vi "水样测试.vi"(11 "数据标记表":string(combo)="N") -> ()   [LabVIEW 2016, in "斯坦道多参数.lvlib"]
panel:
  out "运行状态":u16(ring) items=["空闲", "水样测试", "标样核查"]
  out "多参数运行日志":string
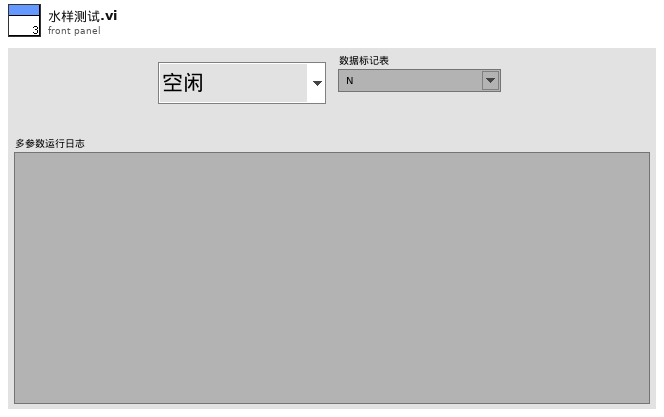
[diagram p1: front panel]
types:
  T1 = typedef "集成多参数单参数字段定义.ctl" = cluster{"时间":timestamp, "测量模式":string, "数据类型":string, "检测值":sgl, "单位":string, "数据标识":string, "信号值":sgl, "标样参考值":sgl, "因子编码":string, "探头温度":sgl, "LastTime":timestamp}
  T2 = cluster{"水温":bool, "pH":bool, "DO":bool, "DOper":bool, "电导率":bool, "ORP":bool, "浊度":bool, "叶绿素a":bool, "藻密度":bool, "COD":bool, "DO2":bool, "DOper":bool, "氯化物":bool, "氨氮":bool, "水中油":bool}
  T3 = cluster{"ph":bool, "DO":bool, "Cond":bool, "Turb":bool, "叶绿素a":bool, "藻密度":bool, "ORP":bool, "cod":bool, "DO2":bool, "氯化物":bool, "氨氮":bool, "水中油":bool}
  T4 = cluster{"温度测量值":sgl, "测量值":sgl, "温度偏移修正值":sgl, "信号值":sgl, "数据标识":string}
  T5 = cluster{"温度测量值":sgl, "DO%":sgl, "DOmg/L":sgl, "温度偏移修正值":sgl, "数据标识mg/L":string, "数据标识%":string}
  T6 = cluster{"CH":u16, "监测值":dbl, "信号值":sgl, "数据标识":string}
  T7 = cluster{"水样数据时间":timestamp, "水温":dbl, "pH":dbl, "DO":dbl, "DOper":dbl, "电导率":dbl, "ORP":dbl, "浊度":dbl, "叶绿素a":dbl, "藻密度":dbl, "COD":dbl, "DO2":dbl, "DO2per":dbl, "氯化物":dbl, "氨氮":dbl, "水中油":dbl}
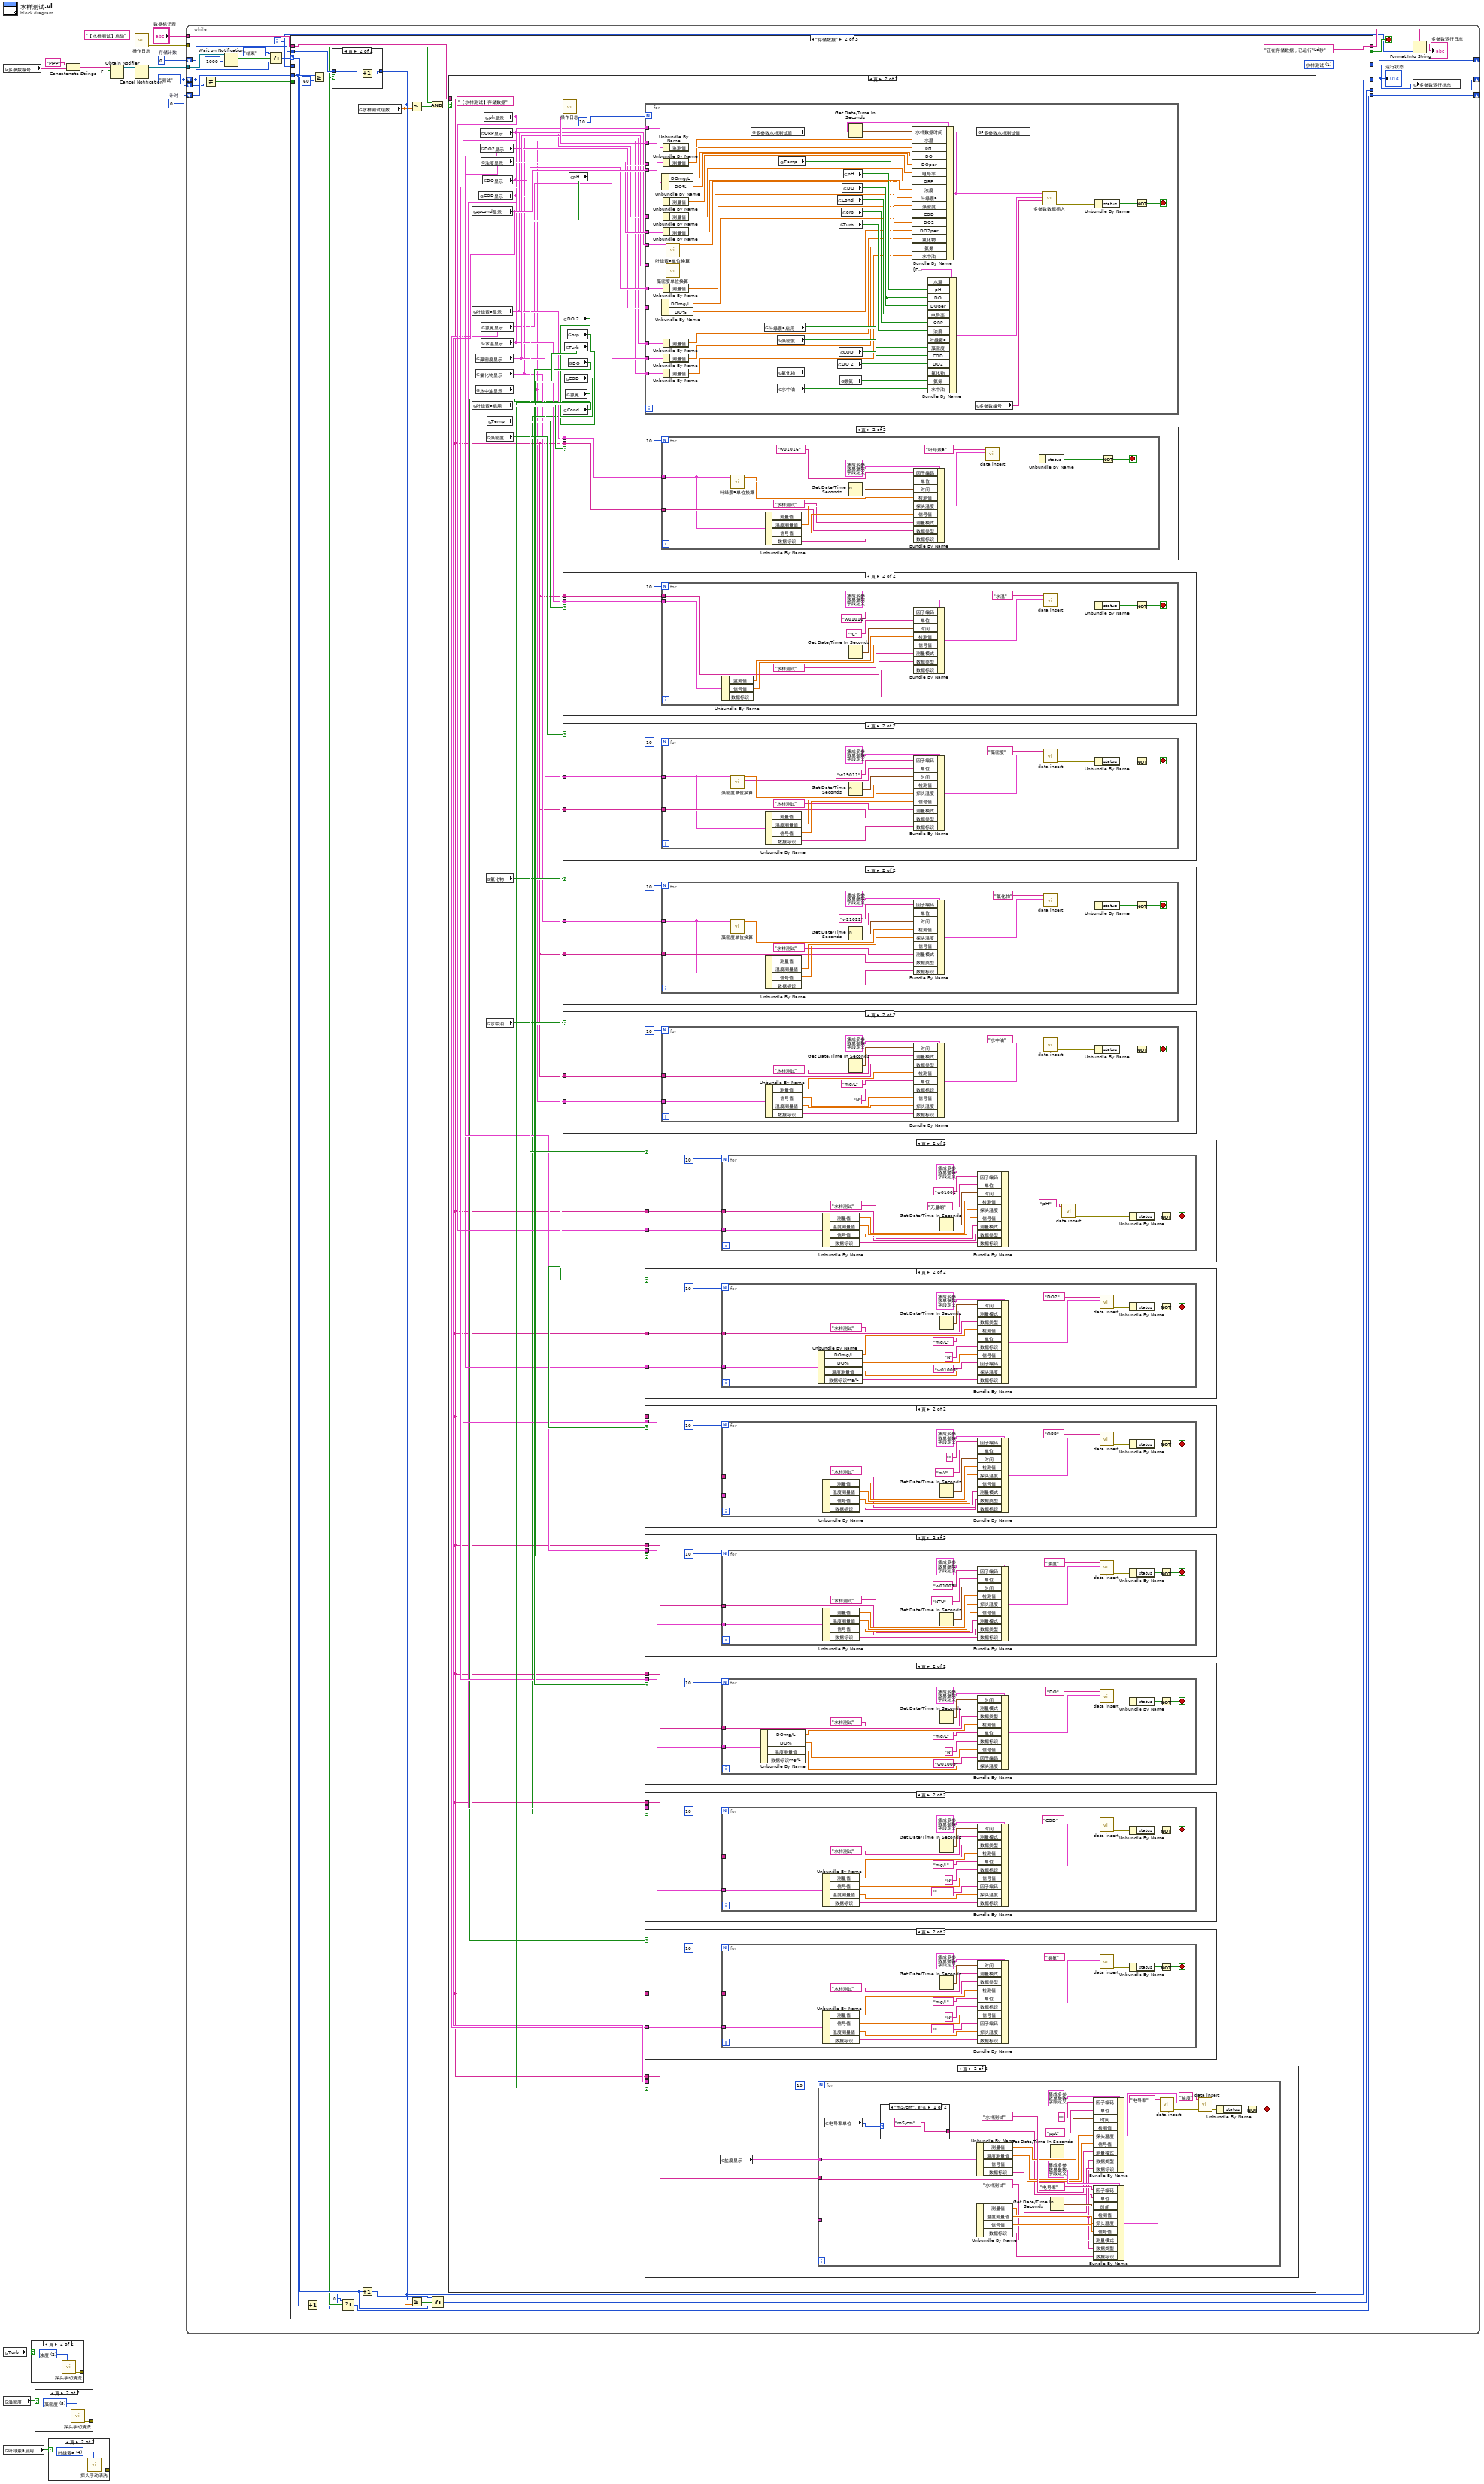
[diagram p0: block diagram]
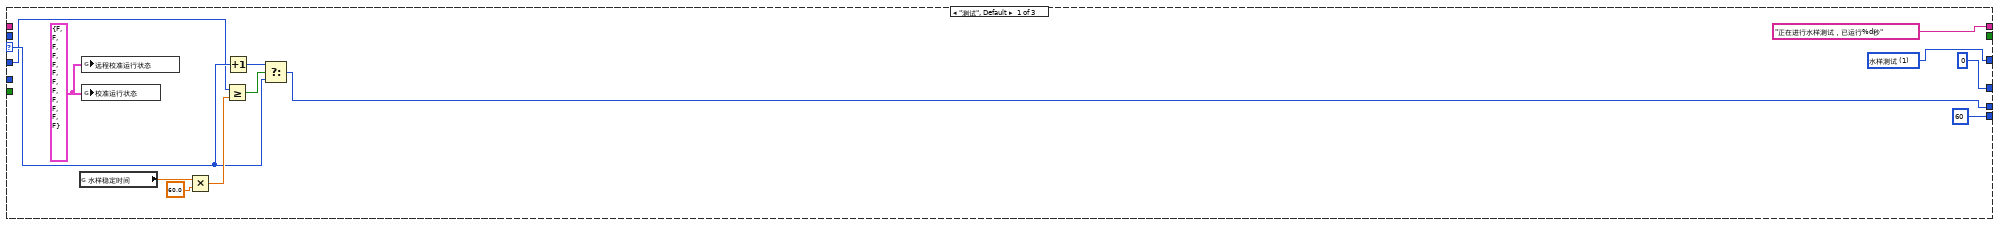
[diagram p5: hidden frame]
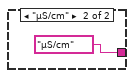
[diagram p18: hidden frame]
diagram:
  w7 = 0  # 存储计数
  w8 = 0  # 计时
  w3 = enum16{"测试", "存储数据", "结束"}."测试" ("枚举")
  n1 = global read "多参数全局变量.vi" "多参数编号"() -> (w9:string)
  n2 = global read "断电保存变量.vi" "Turb"() -> (w6:bool)
  n3 = global read "断电保存变量.vi" "藻密度"() -> (w4:bool)
  n4 = global read "断电保存变量.vi" "叶绿素a启用"() -> (w5:bool)
  n5 = case shown="真" w6 {
    tunnel: [_ w16] -> _
    frame False {
    }
    frame True {
      w17 = u16 2 items=["pH", "DO", "浊度", "电导率", "叶绿素a", "藻密度", "ORP", "DO2"] ("校准参数")
      n6 = call "探头手动清洗.vi"("校准参数"=w17) -> ("error out"=w16:errorcluster)  [unwired: 10 in]
    }
  }
  n7 = case shown="真" w4 {
    tunnel: [_ w18] -> _
    frame False {
    }
    frame True {
      w19 = u16 5 items=["pH", "DO", "浊度", "电导率", "叶绿素a", "藻密度", "ORP", "DO2"] ("校准参数")
      n8 = call "探头手动清洗.vi"("校准参数"=w19) -> ("error out"=w18:errorcluster)  [unwired: 10 in]
    }
  }
  n9 = case shown="真" w5 {
    tunnel: [_ w20] -> _
    frame False {
    }
    frame True {
      w21 = u16 4 items=["pH", "DO", "浊度", "电导率", "叶绿素a", "藻密度", "ORP", "DO2"] ("校准参数")
      n10 = call "探头手动清洗.vi"("校准参数"=w21) -> ("error out"=w20:errorcluster)  [unwired: 10 in]
    }
  }
  n11 = Concatenate Strings("MPP" ("名称（未命名）"), w9) -> (w10:string)
  n12 = Obtain Notifier(name (unnamed)=w10, notification data type=FALSE) -> (notifier out=w13:refnum<notifier>)  [unwired: 2 in, 2 out]
  n13 = call "操作日志.vi"("日志信息"="【水样测试】启动") -> ("error out"=w1:errorcluster)  [unwired: 10 in]
  n14 = Cancel Notification(0:w13) -> (8:w12:refnum<notifier>)  [unwired: 1 in, 2 out]
  n15 = while {
    shift-right: [w26] -> _
    shift-left: w3 -> [w24]
    tunnel: w12 -> [w37]
    tunnel: "数据标记表" -> [w32]
    shift-right: [w28] -> _
    shift-left: w8 -> [w30]
    shift-right: [w27] -> _
    shift-left: w7 -> [w29]
    shift-left: w3 -> [w23]
    tunnel: w1 -> [_]
    i -> [w25]
    stop <- w40 stop-if-true
    n16 = Not Equal?(x=w24, y=w23) -> (x != y?=w22:bool)
    n17 = Wait on Notification(notifier=w37, timeout in ms (-1)=1000 ("超时毫秒(-1)")) -> (notification=w35:bool)  [unwired: 2 in, 3 out]
    n18 = Select(t=enum16{"测试", "存储数据", "结束"}."结束" ("枚举"), s=w35, f=w24) -> (s? t:f=w33:enum16{"测试", "存储数据", "结束"})
    n19 = case shown="\"存储数据\"" w33 {
      selector: w33 -> [w47 w61 _]
      tunnel: [_ _ TRUE] -> w40
      tunnel: ["正在进行水样测试，已运行%d秒" ("格式字符串") "正在存储数据，已运行%d秒" ("格式字符串") "测试停止，累计运行%d秒" ("格式字符串")] -> w39
      tunnel: [w52 w66 w424] -> w31
      tunnel: w32 -> [_ w71 _]
      tunnel: w30 -> [_ w69 _]
      tunnel: w29 -> [_ w70 _]
      tunnel: [60 w54 0] -> w28
      tunnel: [0 w60 0] -> w27
      tunnel: [w45 w64 enum16{"测试", "存储数据", "结束"}."结束" ("枚举")] -> w26
      tunnel: w25 -> [w42 _ _]
      tunnel: w22 -> [_ _ w420]
      frame "测试", Default {
        w41 = T3 {"ph"=FALSE, "DO"=FALSE, "Cond"=FALSE, "Turb"=FALSE, "叶绿素a"=FALSE, "藻密度"=FALSE, "ORP"=FALSE, "cod"=FALSE, "DO2"=FALSE, "氯化物"=FALSE, "氨氮"=FALSE, "水中油"=FALSE} ("远程校准运行状态")
        w52 = u16 1 items=["空闲", "水样测试", "标样核查"] ("多参数运行状态")
        n20 = global read "断电保存变量.vi" "水样稳定时间"() -> (w51:dbl)
        n21 = global write "多参数全局变量.vi" "远程校准运行状态"(w41) -> ()
        n22 = global write "多参数全局变量.vi" "校准运行状态"(w41) -> ()
        n23 = Multiply(x=w51, y=60.0) -> (x*y=w49:dbl)
        n24 = Greater Or Equal?(x=w42, y=w49) -> (x >= y?=w48:bool)
        n25 = Increment(x=w47) -> (x+1=w46:enum16{"测试", "存储数据", "结束"})
        n26 = Select(t=w46, s=w48, f=w47) -> (s? t:f=w45:enum16{"测试", "存储数据", "结束"})
      }
      frame "存储数据" {
        w66 = u16 1 items=["空闲", "水样测试", "标样核查"] ("多参数运行状态")
        n27 = Increment(x=w69) -> (x+1=w56:i32)
        n28 = Greater Or Equal?(x=w69, y=60) -> (x >= y?=w57:bool)
        n29 = case shown="真" w57 {
          tunnel: w70 -> [w72 w74]
          tunnel: [w72 w73] -> w60
          frame False {
          }
          frame True {
            n30 = Increment(x=w74) -> (x+1=w73:i32)
          }
        }
        n31 = Select(t=0, s=w57, f=w56) -> (s? t:f=w54:i32)
        n32 = global read "断电保存变量.vi" "水样测试组数"() -> (w59:dbl)
        n33 = Increment(x=w61) -> (x+1=w62:enum16{"测试", "存储数据", "结束"})
        n34 = Less Or Equal?(x=w60, y=w59) -> (x <= y?=w65:bool)
        n35 = Greater Or Equal?(x=w60, y=w59) -> (x >= y?=w58:bool)
        n36 = And(x=w57, y=w65) -> (x .and. y?=w63:bool)
        n37 = Select(t=w62, s=w58, f=w61) -> (s? t:f=w64:enum16{"测试", "存储数据", "结束"})
        n38 = case shown="真" w63 {
          tunnel: w71 -> [_ w76]
          frame False {
          }
          frame True {
            n39 = global read "多参数全局变量.vi" "spcond显示"() -> (w94:T4)
            n40 = global read "多参数全局变量.vi" "叶绿素a显示"() -> (w88:T4)
            n41 = global read "断电保存变量.vi" "叶绿素a启用"() -> (w103:bool)
            n42 = global read "多参数全局变量.vi" "藻密度显示"() -> (w90:T4)
            n43 = global read "多参数全局变量.vi" "氯化物显示"() -> (w80:T4)
            n44 = global read "多参数全局变量.vi" "水中油显示"() -> (w75:T4)
            n45 = global read "多参数全局变量.vi" "COD显示"() -> (w85:T4)
            n46 = global read "多参数全局变量.vi" "ORP显示"() -> (w87:T4)
            n47 = global read "多参数全局变量.vi" "DO2显示"() -> (w82:T5)
            n48 = global read "多参数全局变量.vi" "浊度显示"() -> (w92:T4)
            n49 = global read "多参数全局变量.vi" "氨氮显示"() -> (w78:T4)
            n50 = global read "多参数全局变量.vi" "水温显示"() -> (w89:T6)
            n51 = global read "多参数全局变量.vi" "DO显示"() -> (w91:T5)
            n52 = global read "多参数全局变量.vi" "ph显示"() -> (w93:T4)
            n53 = global read "断电保存变量.vi" "藻密度"() -> (w97:bool)
            n54 = global read "断电保存变量.vi" "氯化物"() -> (w81:bool)
            n55 = global read "断电保存变量.vi" "水中油"() -> (w77:bool)
            n56 = global read "断电保存变量.vi" "Temp"() -> (w98:bool)
            n57 = call "操作日志.vi"("日志信息"="【水样测试】存储数据") -> ()  [unwired: 10 in, 1 out]
            n58 = global read "断电保存变量.vi" "DO 2"() -> (w83:bool)
            n59 = global read "断电保存变量.vi" "Cond"() -> (w101:bool)
            n60 = case shown="真" w103 {
              tunnel: w76 -> [_ w292]
              tunnel: w88 -> [_ w290]
              frame False {
              }
              frame True {
                n61 = for {
                  N: 10 -> [_]
                  tunnel: w292 -> [w298]
                  tunnel: w290 -> [w295]
                  stop <- w302 stop-if-true
                  n62 = call "叶绿素a单位换算.vi"("叶绿素a显示"=w295) -> ("检测值1.单位"=w294:string, "测量值"=w293:sgl)  [unwired: 8 in, 1 out]
                  n63 = Unbundle By Name(w295) -> ("温度测量值"=w308:sgl, "信号值"=w301:sgl, "数据标识"=w297:string)  [unwired: 1 out]
                  n64 = Get Date/Time In Seconds() -> (seconds since 1Jan1904=w300:timestamp)
                  n65 = Bundle By Name(cluster=T1 {"时间"=timestamp(0 s since 1904-01-01), "测量模式"="水样测试", "数据类型"="N", "检测值"=0.0, "单位"="mg/L", "数据标识"="N", "信号值"=0.0, "标样参考值"=0.0, "因子编码"="", "探头温度"=0.0, "LastTime"=timestamp(0 s since 1904-01-01)} ("data"), "因子编码"="w01016", "单位"=w294, "时间"=w300, "检测值"=w293, "探头温度"=w308, "信号值"=w301, "测量模式"="水样测试", "数据类型"=w298, "数据标识"=w297) -> (w306:T1)
                  n66 = call "data insert.vi"("data"=w306, "table in"="叶绿素a" ("table输入")) -> ("error out"=w304:errorcluster)  [unwired: 9 in]
                  n67 = Unbundle By Name(w304) -> ("status"=w303:bool)
                  n68 = Not(x=w303) -> (.not. x?=w302:bool)
                }
              }
            }
            n69 = case shown="真" w98 {
              tunnel: w76 -> [_ w404]
              tunnel: w89 -> [_ w402]
              frame False {
              }
              frame True {
                n70 = for {
                  N: 10 -> [_]
                  tunnel: w404 -> [w408]
                  tunnel: w402 -> [w407]
                  stop <- w412 stop-if-true
                  n71 = Unbundle By Name(w407) -> ("监测值"=w415:dbl, "信号值"=w410:sgl, "数据标识"=w406:string)
                  n72 = Get Date/Time In Seconds() -> (seconds since 1Jan1904=w411:timestamp)
                  n73 = Bundle By Name(cluster=T1 {"时间"=timestamp(0 s since 1904-01-01), "测量模式"="水样测试", "数据类型"="N", "检测值"=0.0, "单位"="mg/L", "数据标识"="N", "信号值"=0.0, "标样参考值"=0.0, "因子编码"="", "探头温度"=0.0, "LastTime"=timestamp(0 s since 1904-01-01)} ("data"), "因子编码"="w01010", "单位"="℃", "时间"=w411, "检测值"=w415, "信号值"=w410, "测量模式"="水样测试", "数据类型"=w408, "数据标识"=w406) -> (w418:T1)
                  n74 = call "data insert.vi"("data"=w418, "table in"="水温" ("table输入")) -> ("error out"=w414:errorcluster)  [unwired: 9 in]
                  n75 = Unbundle By Name(w414) -> ("status"=w413:bool)
                  n76 = Not(x=w413) -> (.not. x?=w412:bool)
                }
              }
            }
            n77 = case shown="真" w97 {
              tunnel: w76 -> [_ w273]
              tunnel: w90 -> [_ w271]
              frame False {
              }
              frame True {
                n78 = for {
                  N: 10 -> [_]
                  tunnel: w273 -> [w280]
                  tunnel: w271 -> [w276]
                  stop <- w281 stop-if-true
                  n79 = call "藻密度单位换算.vi"("藻密度显示"=w276) -> ("检测值1.单位"=w274:string, "测量值"=w275:sgl)  [unwired: 8 in, 1 out]
                  n80 = Unbundle By Name(w276) -> ("温度测量值"=w289:sgl, "信号值"=w282:sgl, "数据标识"=w278:string)  [unwired: 1 out]
                  n81 = Get Date/Time In Seconds() -> (seconds since 1Jan1904=w283:timestamp)
                  n82 = Bundle By Name(cluster=T1 {"时间"=timestamp(0 s since 1904-01-01), "测量模式"="水样测试", "数据类型"="N", "检测值"=0.0, "单位"="mg/L", "数据标识"="N", "信号值"=0.0, "标样参考值"=0.0, "因子编码"="", "探头温度"=0.0, "LastTime"=timestamp(0 s since 1904-01-01)} ("data"), "因子编码"="w19011", "单位"=w274, "时间"=w283, "检测值"=w275, "探头温度"=w289, "信号值"=w282, "测量模式"="水样测试", "数据类型"=w280, "数据标识"=w278) -> (w284:T1)
                  n83 = call "data insert.vi"("data"=w284, "table in"="藻密度" ("table输入")) -> ("error out"=w286:errorcluster)  [unwired: 9 in]
                  n84 = Unbundle By Name(w286) -> ("status"=w285:bool)
                  n85 = Not(x=w285) -> (.not. x?=w281:bool)
                }
              }
            }
            n86 = case shown="真" w81 {
              tunnel: w76 -> [_ w145]
              tunnel: w80 -> [_ w143]
              frame False {
              }
              frame True {
                n87 = for {
                  N: 10 -> [_]
                  tunnel: w145 -> [w154]
                  tunnel: w143 -> [w150]
                  stop <- w155 stop-if-true
                  n88 = call "藻密度单位换算.vi"("藻密度显示"=w150) -> ("检测值1.单位"=w148:string, "测量值"=w149:sgl)  [unwired: 8 in, 1 out]
                  n89 = Unbundle By Name(w150) -> ("温度测量值"=w161:sgl, "信号值"=w156:sgl, "数据标识"=w152:string)  [unwired: 1 out]
                  n90 = Get Date/Time In Seconds() -> (seconds since 1Jan1904=w157:timestamp)
                  n91 = Bundle By Name(cluster=T1 {"时间"=timestamp(0 s since 1904-01-01), "测量模式"="水样测试", "数据类型"="N", "检测值"=0.0, "单位"="mg/L", "数据标识"="N", "信号值"=0.0, "标样参考值"=0.0, "因子编码"="", "探头温度"=0.0, "LastTime"=timestamp(0 s since 1904-01-01)} ("data"), "因子编码"="w21022", "单位"=w148, "时间"=w157, "检测值"=w149, "探头温度"=w161, "信号值"=w156, "测量模式"="水样测试", "数据类型"=w154, "数据标识"=w152) -> (w158:T1)
                  n92 = call "data insert.vi"("data"=w158, "table in"="氯化物") -> ("error out"=w160:errorcluster)  [unwired: 9 in]
                  n93 = Unbundle By Name(w160) -> ("status"=w159:bool)
                  n94 = Not(x=w159) -> (.not. x?=w155:bool)
                }
              }
            }
            n95 = case shown="真" w77 {
              tunnel: w76 -> [_ w106]
              tunnel: w75 -> [_ w104]
              frame False {
              }
              frame True {
                n96 = for {
                  N: 10 -> [_]
                  tunnel: w106 -> [w119]
                  tunnel: w104 -> [w112]
                  stop <- w122 stop-if-true
                  n97 = Unbundle By Name(w112) -> ("测量值"=w111:sgl, "信号值"=w110:sgl, "温度测量值"=w109:sgl, "数据标识"=w108:string)
                  n98 = Get Date/Time In Seconds() -> (seconds since 1Jan1904=w121:timestamp)
                  n99 = Bundle By Name(cluster=T1 {"时间"=timestamp(0 s since 1904-01-01), "测量模式"="水样测试", "数据类型"="N", "检测值"=0.0, "单位"="mg/L", "数据标识"="N", "信号值"=0.0, "标样参考值"=0.0, "因子编码"="", "探头温度"=0.0, "LastTime"=timestamp(0 s since 1904-01-01)} ("data"), "时间"=w121, "测量模式"="水样测试", "数据类型"=w119, "检测值"=w111, "单位"="mg/L", "数据标识"="N" ("水样数据标识"), "信号值"=w110, "探头温度"=w109, "数据标识"=w108) -> (w114:T1)
                  n100 = call "data insert.vi"("data"=w114, "table in"="水中油") -> ("error out"=w115:errorcluster)  [unwired: 9 in]
                  n101 = Unbundle By Name(w115) -> ("status"=w116:bool)
                  n102 = Not(x=w116) -> (.not. x?=w122:bool)
                }
              }
            }
            n103 = global read "断电保存变量.vi" "Turb"() -> (w102:bool)
            n104 = global read "断电保存变量.vi" "COD"() -> (w84:bool)
            n105 = global read "断电保存变量.vi" "氨氮"() -> (w79:bool)
            n106 = global read "断电保存变量.vi" "orp"() -> (w96:bool)
            n107 = global read "断电保存变量.vi" "DO"() -> (w100:bool)
            n108 = global read "断电保存变量.vi" "pH"() -> (w99:bool)
            n109 = for {
              N: 10 -> [_]
              tunnel: w89 -> [w231]
              tunnel: w93 -> [w230]
              tunnel: w91 -> [w229]
              tunnel: w94 -> [w228]
              tunnel: w87 -> [w227]
              tunnel: w92 -> [w226]
              tunnel: w88 -> [w216]
              tunnel: w90 -> [w218]
              tunnel: w85 -> [w224]
              tunnel: w82 -> [w221]
              tunnel: w80 -> [w212]
              tunnel: w78 -> [w210]
              tunnel: w75 -> [w203]
              stop <- w233 stop-if-true
              n110 = Unbundle By Name(w229) -> ("DOmg/L"=w248:sgl, "DO%"=w247:sgl)
              n111 = Unbundle By Name(w221) -> ("DOmg/L"=w220:sgl, "DO%"=w219:sgl)
              n112 = Unbundle By Name(w231) -> ("监测值"=w250:dbl)
              n113 = Unbundle By Name(w230) -> ("测量值"=w249:sgl)
              n114 = Unbundle By Name(w228) -> ("测量值"=w246:sgl)
              n115 = Unbundle By Name(w227) -> ("测量值"=w245:sgl)
              n116 = Unbundle By Name(w226) -> ("测量值"=w244:sgl)
              n117 = Unbundle By Name(w224) -> ("测量值"=w223:sgl)
              n118 = Unbundle By Name(w212) -> ("测量值"=w211:sgl)
              n119 = Unbundle By Name(w210) -> ("测量值"=w209:sgl)
              n120 = Unbundle By Name(w203) -> ("测量值"=w202:sgl)
              n121 = call "叶绿素a单位换算.vi"("叶绿素a显示"=w216) -> ("测量值"=w215:sgl)  [unwired: 8 in, 2 out]
              n122 = call "藻密度单位换算.vi"("藻密度显示"=w218) -> ("测量值"=w217:sgl)  [unwired: 8 in, 2 out]
              n123 = global read "多参数全局变量.vi" "多参数水样测试值"() -> (w207:T7)
              n124 = global read "断电保存变量.vi" "叶绿素a启用"() -> (w237:bool)
              n125 = global read "断电保存变量.vi" "藻密度"() -> (w240:bool)
              n126 = global read "断电保存变量.vi" "氯化物"() -> (w213:bool)
              n127 = global read "断电保存变量.vi" "水中油"() -> (w204:bool)
              n128 = global read "断电保存变量.vi" "Temp"() -> (w239:bool)
              n129 = global read "断电保存变量.vi" "Cond"() -> (w242:bool)
              n130 = global read "断电保存变量.vi" "DO 2"() -> (w222:bool)
              n131 = global read "断电保存变量.vi" "Turb"() -> (w241:bool)
              n132 = global read "断电保存变量.vi" "COD"() -> (w225:bool)
              n133 = global read "断电保存变量.vi" "氨氮"() -> (w208:bool)
              n134 = global read "断电保存变量.vi" "orp"() -> (w238:bool)
              n135 = global read "断电保存变量.vi" "DO"() -> (w236:bool)
              n136 = global read "断电保存变量.vi" "pH"() -> (w243:bool)
              n137 = Get Date/Time In Seconds() -> (seconds since 1Jan1904=w251:timestamp)
              n138 = Bundle By Name(cluster=w207, "水样数据时间"=w251, "水温"=w250, "pH"=w249, "DO"=w248, "DOper"=w247, "电导率"=w246, "ORP"=w245, "浊度"=w244, "叶绿素a"=w215, "藻密度"=w217, "COD"=w223, "DO2"=w220, "DO2per"=w219, "氯化物"=w211, "氨氮"=w209, "水中油"=w202) -> (w214:T7)
              n139 = Bundle By Name(cluster=T2 {"水温"=FALSE, "pH"=FALSE, "DO"=FALSE, "DOper"=FALSE, "电导率"=FALSE, "ORP"=FALSE, "浊度"=FALSE, "叶绿素a"=FALSE, "藻密度"=FALSE, "COD"=FALSE, "DO2"=FALSE, "DOper"=FALSE, "氯化物"=FALSE, "氨氮"=FALSE, "水中油"=FALSE} ("columns enable"), "水温"=w239, "pH"=w243, "DO"=w236, "DOper"=w236, "电导率"=w242, "ORP"=w238, "浊度"=w241, "叶绿素a"=w237, "藻密度"=w240, "COD"=w225, "DO2"=w222, "氯化物"=w213, "氨氮"=w208, "水中油"=w204) -> (w205:T2)
              n140 = global read "多参数全局变量.vi" "多参数编号"() -> (w232:string)
              n141 = global write "多参数全局变量.vi" "多参数水样测试值"(w214) -> ()
              n142 = call "多参数数据插入.vi"("编号"=w232, "columns enable"=w205, "data in"=w214) -> ("error out"=w235:errorcluster)  [unwired: 8 in]
              n143 = Unbundle By Name(w235) -> ("status"=w234:bool)
              n144 = Not(x=w234) -> (.not. x?=w233:bool)
            }
            n145 = case shown="真" w99 {
              tunnel: w76 -> [_ w385]
              tunnel: w93 -> [_ w383]
              frame False {
              }
              frame True {
                n146 = for {
                  N: 10 -> [_]
                  tunnel: w385 -> [w389]
                  tunnel: w383 -> [w388]
                  stop <- w393 stop-if-true
                  n147 = Unbundle By Name(w388) -> ("测量值"=w397:sgl, "温度测量值"=w396:sgl, "信号值"=w391:sgl, "数据标识"=w387:string)
                  n148 = Get Date/Time In Seconds() -> (seconds since 1Jan1904=w392:timestamp)
                  n149 = Bundle By Name(cluster=T1 {"时间"=timestamp(0 s since 1904-01-01), "测量模式"="水样测试", "数据类型"="N", "检测值"=0.0, "单位"="mg/L", "数据标识"="N", "信号值"=0.0, "标样参考值"=0.0, "因子编码"="", "探头温度"=0.0, "LastTime"=timestamp(0 s since 1904-01-01)} ("data"), "因子编码"="w01001", "单位"="无量纲", "时间"=w392, "检测值"=w397, "探头温度"=w396, "信号值"=w391, "测量模式"="水样测试", "数据类型"=w389, "数据标识"=w387) -> (w401:T1)
                  n150 = call "data insert.vi"("data"=w401, "table in"="pH" ("table输入")) -> ("error out"=w395:errorcluster)  [unwired: 9 in]
                  n151 = Unbundle By Name(w395) -> ("status"=w394:bool)
                  n152 = Not(x=w394) -> (.not. x?=w393:bool)
                }
              }
            }
            n153 = case shown="真" w83 {
              tunnel: w76 -> [_ w164]
              tunnel: w82 -> [_ w162]
              frame False {
              }
              frame True {
                n154 = for {
                  N: 10 -> [_]
                  tunnel: w164 -> [w178]
                  tunnel: w162 -> [w168]
                  stop <- w181 stop-if-true
                  n155 = Unbundle By Name(w168) -> ("DOmg/L"=w177:sgl, "DO%"=w170:sgl, "温度测量值"=w171:sgl, "数据标识mg/L"=w167:string)
                  n156 = Get Date/Time In Seconds() -> (seconds since 1Jan1904=w180:timestamp)
                  n157 = Bundle By Name(cluster=T1 {"时间"=timestamp(0 s since 1904-01-01), "测量模式"="水样测试", "数据类型"="N", "检测值"=0.0, "单位"="mg/L", "数据标识"="N", "信号值"=0.0, "标样参考值"=0.0, "因子编码"="", "探头温度"=0.0, "LastTime"=timestamp(0 s since 1904-01-01)} ("data"), "时间"=w180, "测量模式"="水样测试", "数据类型"=w178, "检测值"=w177, "单位"="mg/L", "数据标识"="N" ("水样数据标识"), "信号值"=w170, "因子编码"="w01009", "探头温度"=w171, "数据标识"=w167) -> (w169:T1)
                  n158 = call "data insert.vi"("data"=w169, "table in"="DO2") -> ("error out"=w173:errorcluster)  [unwired: 9 in]
                  n159 = Unbundle By Name(w173) -> ("status"=w174:bool)
                  n160 = Not(x=w174) -> (.not. x?=w181:bool)
                }
              }
            }
            n161 = case shown="真" w96 {
              tunnel: w76 -> [_ w254]
              tunnel: w87 -> [_ w252]
              frame False {
              }
              frame True {
                n162 = for {
                  N: 10 -> [_]
                  tunnel: w254 -> [w260]
                  tunnel: w252 -> [w258]
                  stop <- w263 stop-if-true
                  n163 = Unbundle By Name(w258) -> ("测量值"=w270:sgl, "温度测量值"=w268:sgl, "信号值"=w261:sgl, "数据标识"=w257:string)
                  n164 = Get Date/Time In Seconds() -> (seconds since 1Jan1904=w262:timestamp)
                  n165 = Bundle By Name(cluster=T1 {"时间"=timestamp(0 s since 1904-01-01), "测量模式"="水样测试", "数据类型"="N", "检测值"=0.0, "单位"="mg/L", "数据标识"="N", "信号值"=0.0, "标样参考值"=0.0, "因子编码"="", "探头温度"=0.0, "LastTime"=timestamp(0 s since 1904-01-01)} ("data"), "因子编码"="", "单位"="mV", "时间"=w262, "检测值"=w270, "探头温度"=w268, "信号值"=w261, "测量模式"="水样测试", "数据类型"=w260, "数据标识"=w257) -> (w255:T1)
                  n166 = call "data insert.vi"("data"=w255, "table in"="ORP" ("table输入")) -> ("error out"=w266:errorcluster)  [unwired: 9 in]
                  n167 = Unbundle By Name(w266) -> ("status"=w265:bool)
                  n168 = Not(x=w265) -> (.not. x?=w263:bool)
                }
              }
            }
            n169 = case shown="真" w102 {
              tunnel: w76 -> [_ w311]
              tunnel: w92 -> [_ w309]
              frame False {
              }
              frame True {
                n170 = for {
                  N: 10 -> [_]
                  tunnel: w311 -> [w315]
                  tunnel: w309 -> [w314]
                  stop <- w319 stop-if-true
                  n171 = Unbundle By Name(w314) -> ("测量值"=w323:sgl, "温度测量值"=w322:sgl, "信号值"=w317:sgl, "数据标识"=w313:string)
                  n172 = Get Date/Time In Seconds() -> (seconds since 1Jan1904=w318:timestamp)
                  n173 = Bundle By Name(cluster=T1 {"时间"=timestamp(0 s since 1904-01-01), "测量模式"="水样测试", "数据类型"="N", "检测值"=0.0, "单位"="mg/L", "数据标识"="N", "信号值"=0.0, "标样参考值"=0.0, "因子编码"="", "探头温度"=0.0, "LastTime"=timestamp(0 s since 1904-01-01)} ("data"), "因子编码"="w01003", "单位"="NTU", "时间"=w318, "检测值"=w323, "探头温度"=w322, "信号值"=w317, "测量模式"="水样测试", "数据类型"=w315, "数据标识"=w313) -> (w326:T1)
                  n174 = call "data insert.vi"("data"=w326, "table in"="浊度" ("table输入")) -> ("error out"=w321:errorcluster)  [unwired: 9 in]
                  n175 = Unbundle By Name(w321) -> ("status"=w320:bool)
                  n176 = Not(x=w320) -> (.not. x?=w319:bool)
                }
              }
            }
            n177 = case shown="真" w100 {
              tunnel: w76 -> [_ w366]
              tunnel: w91 -> [_ w364]
              frame False {
              }
              frame True {
                n178 = for {
                  N: 10 -> [_]
                  tunnel: w366 -> [w378]
                  tunnel: w364 -> [w369]
                  stop <- w382 stop-if-true
                  n179 = Unbundle By Name(w369) -> ("DOmg/L"=w377:sgl, "DO%"=w371:sgl, "温度测量值"=w372:sgl)  [unwired: 1 out]
                  n180 = Get Date/Time In Seconds() -> (seconds since 1Jan1904=w380:timestamp)
                  n181 = Bundle By Name(cluster=T1 {"时间"=timestamp(0 s since 1904-01-01), "测量模式"="水样测试", "数据类型"="N", "检测值"=0.0, "单位"="mg/L", "数据标识"="N", "信号值"=0.0, "标样参考值"=0.0, "因子编码"="", "探头温度"=0.0, "LastTime"=timestamp(0 s since 1904-01-01)} ("data"), "时间"=w380, "测量模式"="水样测试", "数据类型"=w378, "检测值"=w377, "单位"="mg/L", "数据标识"="N", "信号值"=w371, "因子编码"="w01009", "探头温度"=w372) -> (w370:T1)
                  n182 = call "data insert.vi"("data"=w370, "table in"="DO") -> ("error out"=w374:errorcluster)  [unwired: 9 in]
                  n183 = Unbundle By Name(w374) -> ("status"=w375:bool)
                  n184 = Not(x=w375) -> (.not. x?=w382:bool)
                }
              }
            }
            n185 = case shown="真" w84 {
              tunnel: w76 -> [_ w184]
              tunnel: w85 -> [_ w182]
              frame False {
              }
              frame True {
                n186 = for {
                  N: 10 -> [_]
                  tunnel: w184 -> [w197]
                  tunnel: w182 -> [w187]
                  stop <- w201 stop-if-true
                  n187 = Unbundle By Name(w187) -> ("测量值"=w196:sgl, "信号值"=w189:sgl, "温度测量值"=w190:sgl, "数据标识"=w186:string)
                  n188 = Get Date/Time In Seconds() -> (seconds since 1Jan1904=w199:timestamp)
                  n189 = Bundle By Name(cluster=T1 {"时间"=timestamp(0 s since 1904-01-01), "测量模式"="水样测试", "数据类型"="N", "检测值"=0.0, "单位"="mg/L", "数据标识"="N", "信号值"=0.0, "标样参考值"=0.0, "因子编码"="", "探头温度"=0.0, "LastTime"=timestamp(0 s since 1904-01-01)} ("data"), "时间"=w199, "测量模式"="水样测试", "数据类型"=w197, "检测值"=w196, "单位"="mg/L", "数据标识"="N" ("水样数据标识"), "信号值"=w189, "因子编码"="", "探头温度"=w190, "数据标识"=w186) -> (w188:T1)
                  n190 = call "data insert.vi"("data"=w188, "table in"="COD") -> ("error out"=w192:errorcluster)  [unwired: 9 in]
                  n191 = Unbundle By Name(w192) -> ("status"=w193:bool)
                  n192 = Not(x=w193) -> (.not. x?=w201:bool)
                }
              }
            }
            n193 = case shown="真" w79 {
              tunnel: w76 -> [_ w125]
              tunnel: w78 -> [_ w123]
              frame False {
              }
              frame True {
                n194 = for {
                  N: 10 -> [_]
                  tunnel: w125 -> [w138]
                  tunnel: w123 -> [w130]
                  stop <- w142 stop-if-true
                  n195 = Unbundle By Name(w130) -> ("测量值"=w129:sgl, "信号值"=w128:sgl, "温度测量值"=w127:sgl, "数据标识"=w126:string)
                  n196 = Get Date/Time In Seconds() -> (seconds since 1Jan1904=w140:timestamp)
                  n197 = Bundle By Name(cluster=T1 {"时间"=timestamp(0 s since 1904-01-01), "测量模式"="水样测试", "数据类型"="N", "检测值"=0.0, "单位"="mg/L", "数据标识"="N", "信号值"=0.0, "标样参考值"=0.0, "因子编码"="", "探头温度"=0.0, "LastTime"=timestamp(0 s since 1904-01-01)} ("data"), "时间"=w140, "测量模式"="水样测试", "数据类型"=w138, "检测值"=w129, "单位"="mg/L", "数据标识"="N" ("水样数据标识"), "信号值"=w128, "因子编码"="", "探头温度"=w127, "数据标识"=w126) -> (w132:T1)
                  n198 = call "data insert.vi"("data"=w132, "table in"="氨氮") -> ("error out"=w134:errorcluster)  [unwired: 9 in]
                  n199 = Unbundle By Name(w134) -> ("status"=w135:bool)
                  n200 = Not(x=w135) -> (.not. x?=w142:bool)
                }
              }
            }
            n201 = case shown="真" w101 {
              tunnel: w76 -> [_ w331]
              tunnel: w94 -> [_ w329]
              frame False {
              }
              frame True {
                n202 = global read "多参数全局变量.vi" "盐度显示"() -> (w328:T4)
                n203 = for {
                  N: 10 -> [_]
                  tunnel: w331 -> [w339]
                  tunnel: w329 -> [w351]
                  tunnel: w328 -> [w338]
                  stop <- w356 stop-if-true
                  n204 = global read "多参数断电保存全局变量.vi" "电导率单位"() -> (w333:enum16{"mS/cm", "μS/cm"})
                  n205 = case shown="\"mS/cm\", 默认" w333 {
                    tunnel: ["mS/cm" ("单位") "μS/cm" ("单位")] -> w332
                    frame "mS/cm", Default {
                    }
                    frame "μS/cm" {
                    }
                  }
                  n206 = Unbundle By Name(w338) -> ("测量值"=w340:sgl, "温度测量值"=w341:sgl, "信号值"=w344:sgl, "数据标识"=w347:string)
                  n207 = Unbundle By Name(w351) -> ("测量值"=w359:sgl, "温度测量值"=w358:sgl, "信号值"=w354:sgl, "数据标识"=w350:string)
                  n208 = Get Date/Time In Seconds() -> (seconds since 1Jan1904=w343:timestamp)
                  n209 = Get Date/Time In Seconds() -> (seconds since 1Jan1904=w355:timestamp)
                  n210 = Bundle By Name(cluster=T1 {"时间"=timestamp(0 s since 1904-01-01), "测量模式"="水样测试", "数据类型"="N", "检测值"=0.0, "单位"="mg/L", "数据标识"="N", "信号值"=0.0, "标样参考值"=0.0, "因子编码"="", "探头温度"=0.0, "LastTime"=timestamp(0 s since 1904-01-01)} ("data"), "因子编码"="", "单位"="ppt", "时间"=w343, "检测值"=w340, "探头温度"=w341, "信号值"=w344, "测量模式"="水样测试", "数据类型"=w339, "数据标识"=w347) -> (w346:T1)
                  n211 = Bundle By Name(cluster=T1 {"时间"=timestamp(0 s since 1904-01-01), "测量模式"="水样测试", "数据类型"="N", "检测值"=0.0, "单位"="mg/L", "数据标识"="N", "信号值"=0.0, "标样参考值"=0.0, "因子编码"="", "探头温度"=0.0, "LastTime"=timestamp(0 s since 1904-01-01)} ("data"), "因子编码"="电导率", "单位"=w332, "时间"=w355, "检测值"=w359, "探头温度"=w358, "信号值"=w354, "测量模式"="水样测试", "数据类型"=w339, "数据标识"=w350) -> (w352:T1)
                  n212 = call "data insert.vi"("data"=w352, "table in"="电导率" ("table输入")) -> ("error out"=w335:errorcluster)  [unwired: 9 in]
                  n213 = call "data insert.vi"("error in (no error)"=w335, "data"=w346, "table in"="盐度") -> ("error out"=w334:errorcluster)  [unwired: 8 in]
                  n214 = Unbundle By Name(w334) -> ("status"=w357:bool)
                  n215 = Not(x=w357) -> (.not. x?=w356:bool)
                }
              }
            }
          }
        }
      }
      frame "结束" {
        w424 = u16 0 items=["空闲", "水样测试", "标样核查"] ("多参数运行状态")
        n216 = case shown="真" w420 {
          frame False {
          }
          frame True {
            n217 = call "操作日志.vi"("日志信息"="【水样测试】结束") -> ()  [unwired: 10 in, 1 out]
          }
        }
      }
    }
    "运行状态" <- w31
    n218 = Format Into String(format string=w39, w25) -> (resulting string=→"多参数运行日志":string)  [unwired: 2 in, 1 out]
    n219 = global write "多参数全局变量.vi" "多参数运行状态"(w31) -> ()
  }
